vi "MQTT-HomeAssistant-Discovery.vi"(0 "TCP Network Connection in":refnum<k5>, 1 "Device":string="cRIO_1", 2 "DeviceName":string="SaunaTemp", 3 "ChannelBase":string="Temp", 4 "ChannelNames":string[](array[string])=["SaunaHeaterTemp", "SaunaRoofTemp", "SaunaBenchTemp", "SaunaFloorTemp"], 5 "error in (no error)":errorcluster, 6 "Publish Meta":cluster{"QoS":T1, "Retain":T2, "DUP":T3}, 7 "MessageTemplate":string[](array[string]), 9 "ConfigPath":string[](array[string])=["homeassistant/sensor/%s/%s%d/config", "homeassistant/sensor/%s/%s%d/config", "homeassistant/sensor/%s/%s%d/config", "homeassistant/sensor/%s/%s%d/config", "homeassistant/binary_sensor/%s/%s%d/config"]) -> (14 "TCP Network Connection out":refnum<k5>, 15 "Topics":string[](array[string]), 19 "error out":errorcluster)   [LabVIEW 2019]
uses:
  LVMQTT-master/Controls/QoS.ctl
  LVMQTT-master/Controls/Retain_Flag.ctl
  LVMQTT-master/Controls/DUP_Flag.ctl
  LVMQTT-master/MQTT_Functions.lvlib
panel:
  out "Array":errorcluster[](array[cluster])
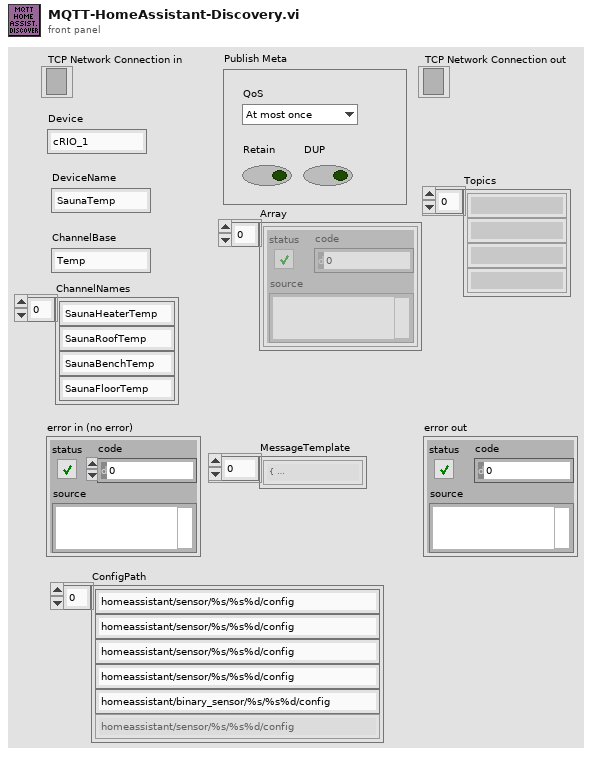
[diagram p1: front panel]
types:
  T1 = typedef "MQTT_Functions.lvlib/QoS.ctl" = enum8{"At most once", "At least once", "Exactly once", "Reserved"}
  T2 = typedef "MQTT_Functions.lvlib/Retain_Flag.ctl" = bool
  T3 = typedef "MQTT_Functions.lvlib/DUP_Flag.ctl" = bool
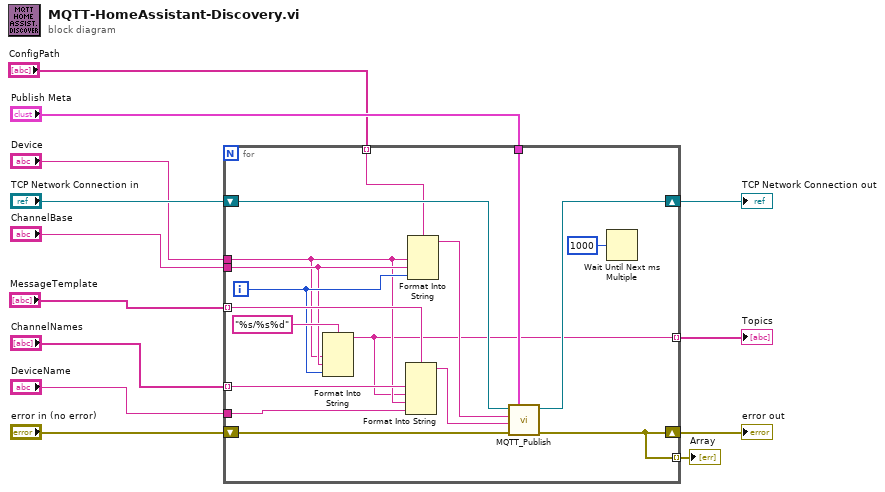
[diagram p0: block diagram]
diagram:
  n1 = for {
    shift-right: [w15] -> w13
    shift-left: "error in (no error)" -> [w30]
    shift-right: [w29] -> w11
    shift-left: "TCP Network Connection in" -> [w28]
    tunnel: "Publish Meta" -> [w27]
    tunnel: "Device" -> [w20]
    tunnel: "ChannelBase" -> [w21]
    tunnel: "MessageTemplate" -> [w25] mode=indexing
    tunnel: "ChannelNames" -> [w24] mode=indexing
    tunnel: "DeviceName" -> [w19]
    tunnel: [w18] -> w3 mode=indexing
    tunnel: [w15] -> w2 mode=indexing
    tunnel: "ConfigPath" -> [w14] mode=indexing
    i -> [w22]
    n2 = Format Into String(format string="%s/%s%d", w20, w21, w22) -> (resulting string=w18:string)  [unwired: 2 in, 1 out]
    n3 = Format Into String(format string=w25, w24, w18, w20, w19) -> (resulting string=w17:string)  [unwired: 2 in, 1 out]
    n4 = Format Into String(format string=w14, w20, w21, w22) -> (resulting string=w26:string)  [unwired: 2 in, 1 out]
    n5 = call "MQTT_Publish.vi"("Publish Meta"=w27, "error in (no error)"=w30, "Message to be published"=w17, "Topic"=w26, "connection ID"=w28) -> ("error out"=w15:errorcluster, "connection ID out"=w29:refnum<k5>)  [unwired: 5 in]
    n6 = Wait Until Next ms Multiple(millisecond multiple=u32 1000) -> ()  [unwired: 1 out]
  }
  "error out" <- w13
  "TCP Network Connection out" <- w11
  "Topics" <- w3
  "Array" <- w2
